vi "互相关.vi"() -> ()   [LabVIEW 2010]
uses:
  <vilib>/Analysis/2dsp.llb/1D Cross Correlation (DBL).vi
  <vilib>/Analysis/NI_AALBase.lvlib
  <vilib>/Analysis/NI_AALPro.lvlib
panel:
  in  "相位":dbl format="%0.2f"
  in  "频率":dbl(slide)=50.0 scale=0.0..200.0
  in  "相位":dbl format="%0.2f"
  in  "频率":dbl(slide)=100.0 scale=0.0..200.0
  in  "时  \n\n标":dbl(knob)=5.600425222700757 scale=0.0..10.0 scale format="%.1f"
  out "互相关函数图形":cluster{dbl, dbl, "Rxx out":dbl[]}(graph)
  in  "stop":bool
  out "示 波  器  图  例":cluster{i32, "时  标":dbl, dbl[][]}(graph)
  # "互 相 关 函 数 实 验"
  # "时 域 信 号"
  # "一   通  道"
  # "二   通  道"
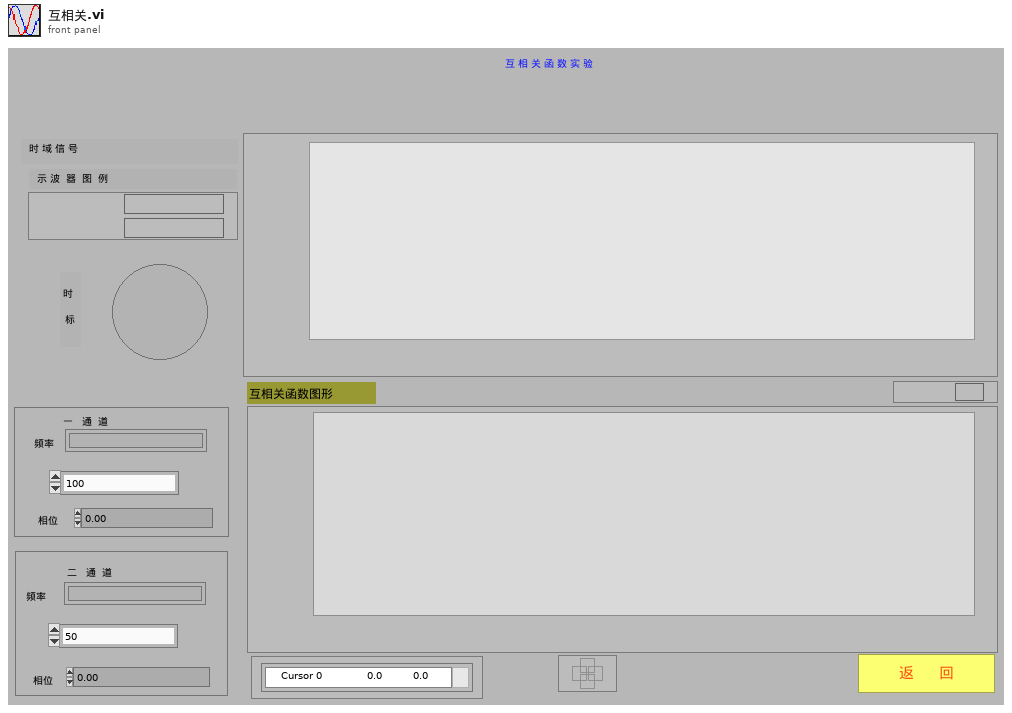
[diagram p1: front panel]
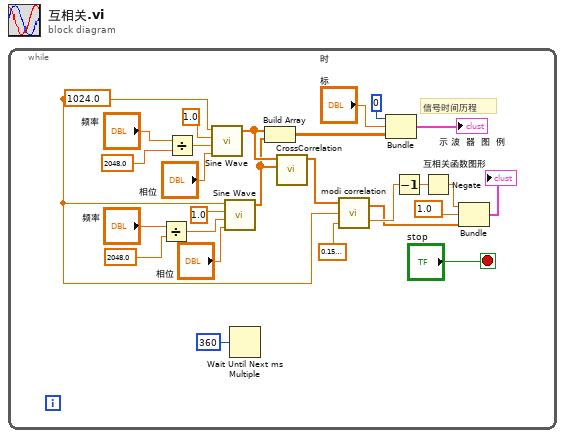
[diagram p0: block diagram]
diagram:
  n1 = while {
    stop <- "stop" stop-if-true
    w12 = 1024.0 ("取样数")
    # "信号时间历程"
    n2 = Divide(x="频率", y=2048.0) -> (x/y=w7:dbl)
    n3 = Divide(x="频率", y=2048.0) -> (x/y=w10:dbl)
    n4 = call <vilib>:"Sine Wave.vi"("samples"=w12, "amplitude"=1.0, "frequency"=w10, "phase in"="相位") -> ("sine wave"=w14:dbl[])  [unwired: 1 in, 2 out]
    n5 = call <vilib>:"Sine Wave.vi"("samples"=w12, "amplitude"=1.0, "frequency"=w7, "phase in"="相位") -> ("sine wave"=w13:dbl[])  [unwired: 1 in, 2 out]
    n6 = Wait Until Next ms Multiple(millisecond multiple=u32 360) -> ()  [unwired: 1 out]
    n7 = Build Array(w14, w13) -> (w24:dbl[][])
    n8 = call-poly <vilib>:"CrossCorrelation.vi"("Y"=w13, "X"=w14) -> ("Rxy"=w23:dbl[])  [unwired: 8 in, 1 out]
    n9 = call "modi correlation.vi"("d"=sgl 0.15, "samples"=w12, "Rxx in"=w23) -> ("n"=w20:dbl, "Rxx out"=w18:dbl[])
    n10 = Bundle(0, "时  \n\n标"="时  \n\n标", w24) -> (→"示 波  器  图  例":cluster{i32, "\n时  \n\n标":dbl, dbl[][]})  [unwired: 1 in]
    n11 = Decrement(x=w20) -> (x-1=w21:dbl)
    n12 = Negate(x=w21) -> (-x=w17:dbl)
    n13 = Bundle(w17, 1.0, "Rxx out"=w18) -> (→"互相关函数图形":cluster{dbl, dbl, "Rxx out ":dbl[]})  [unwired: 1 in]
  }
